vi "Untitled 1.vi"() -> ()   [LabVIEW 2017]
panel:
  out "Free Physical Memory or Largest Contiguous Memory (bytes) 2":i64(graph)
  out "Free Physical Memory or Largest Contiguous Memory (bytes)":dbl(graph)
  in  "stop":bool
  out "size (bytes) 2":i64
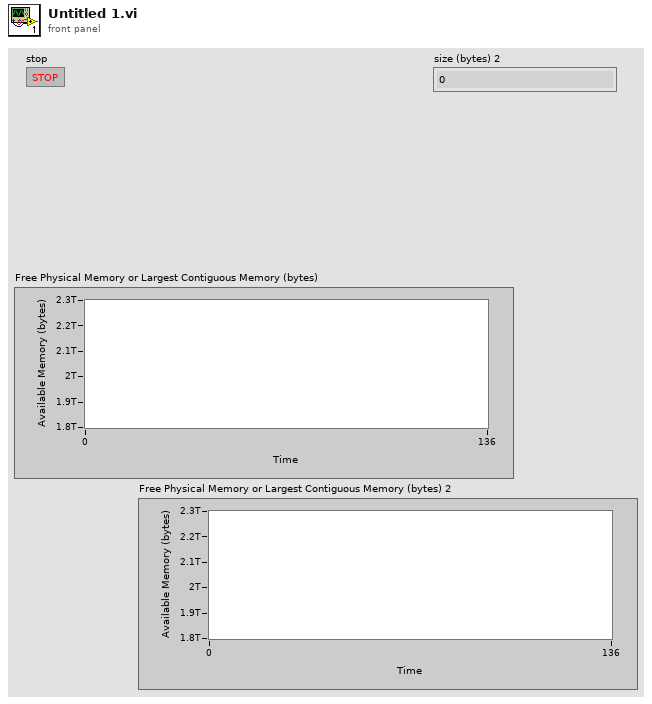
[diagram p1: front panel]
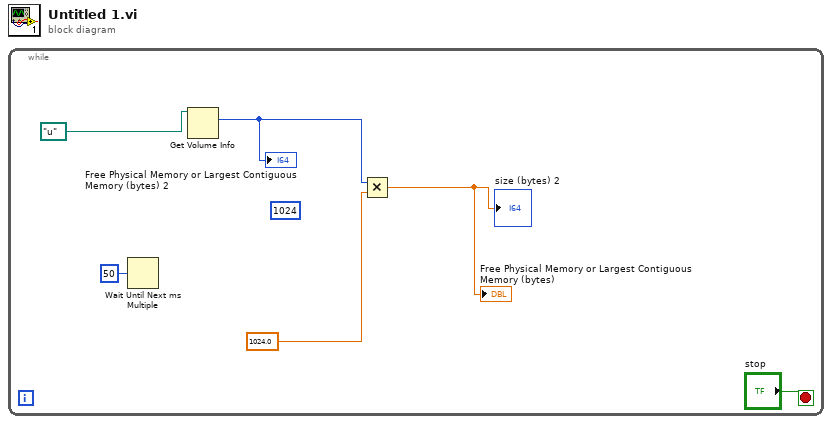
[diagram p0: block diagram]
diagram:
  n1 = while {
    stop <- "stop" stop-if-true
    (unwired) i64 1024 ("y")
    n2 = Wait Until Next ms Multiple(millisecond multiple=u32 50) -> ()  [unwired: 1 out]
    n3 = Get Volume Info(11:path "u:/" ("AVI Path")) -> (2:w1:i64)  [unwired: 1 in, 5 out]
    "Free Physical Memory or Largest Contiguous Memory (bytes) 2" <- w1
    n4 = Multiply(x=w1, y=1024.0 ("x")) -> (x*y=→"size (bytes) 2" →"Free Physical Memory or Largest Contiguous Memory (bytes)":dbl)
  }
